vi "SUB_VI_lettura_messaggio_array.vi"(8 "Errore in ingresso":errorcluster, 11 "TCP Network Connection in":refnum<k5>) -> (0 "Errore in uscita":errorcluster, 2 "Messaggio letto":string, 3 "TCP Network Connection out":refnum<k5>)   [LabVIEW 2023]
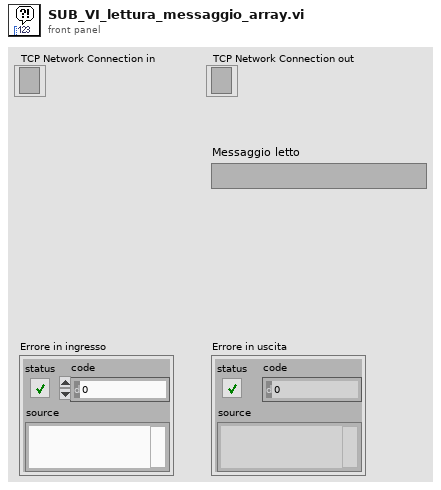
[diagram p1: front panel]
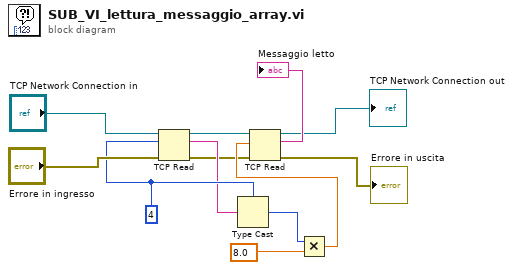
[diagram p0: block diagram]
diagram:
  w4 = 4
  n1 = TCP Read(connection ID="TCP Network Connection in", bytes to read=w4, error in (no error)="Errore in ingresso") -> (connection ID out=w2:refnum<k5>, data out=w3:string, error out=w1:errorcluster)  [unwired: 2 in]
  n2 = Type Cast(type=w4, x=w3) -> (*(type *) &x=w6:i32)
  n3 = Multiply(x=w6, y=8.0) -> (x*y=w7:dbl)
  n4 = TCP Read(connection ID=w2, bytes to read=w7, error in (no error)=w1) -> (connection ID out=→"TCP Network Connection out":refnum<k5>, data out=→"Messaggio letto":string, error out=→"Errore in uscita":errorcluster)  [unwired: 2 in]
